vi "Write Service Name.vi"(8 "error in (no error)":errorcluster, 10 "Service Name":string, 11 "WebSocket Service in":refnum<class "WebSocket Service.lvclass">) -> (0 "error out":errorcluster, 3 "WebSocket Service out":refnum<class "WebSocket Service.lvclass">)   [LabVIEW 2016, in "WebSocket Actors.lvlib" / "WebSocket Service.lvclass"]
uses:
  WebSocket Service.lvclass
  WebSocket Service.lvclass/WebSocket Service.ctl
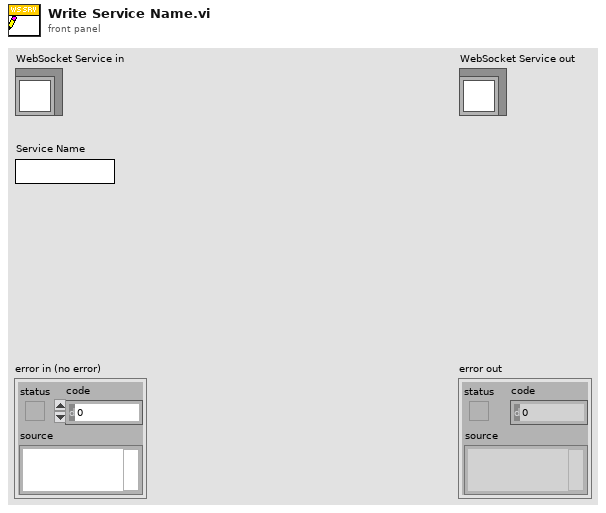
[diagram p1: front panel]
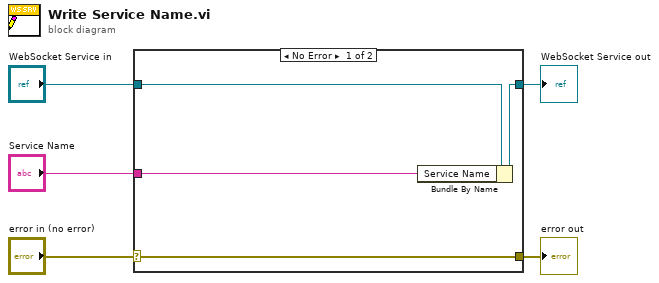
[diagram p0: block diagram]
diagram:
  n1 = case shown="No Error" "error in (no error)" {
    selector: "error in (no error)" -> [w9 w10]
    tunnel: [w9 w10] -> w4
    tunnel: [w7 w11] -> w2
    tunnel: "WebSocket Service in" -> [w8 w11]
    tunnel: "Service Name" -> [w6 _]
    frame No Error {
      n2 = Bundle By Name(cluster=w8, "Service Name"=w6) -> (w7:refnum<class "WebSocket Service.lvclass">)
    }
    frame Error {
    }
  }
  "error out" <- w4
  "WebSocket Service out" <- w2
